vi "Write JSON Variant to File.vi"(8 "Error In":errorcluster, 10 "file (use dialog)":path, 11 "JSON Varaint":variant) -> (0 "error out":errorcluster)   [LabVIEW 2015]
uses:
  <vilib>/addons/_JKI.lib/Serialization/JSON/JKI JSON Serialization.lvlib
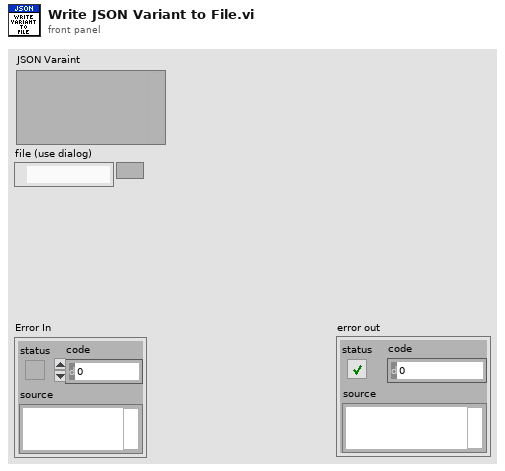
[diagram p1: front panel]
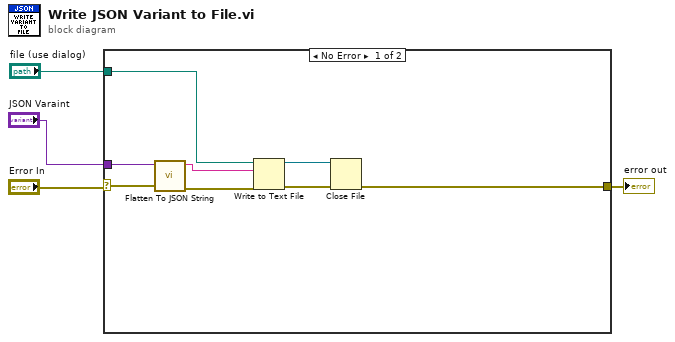
[diagram p0: block diagram]
diagram:
  n1 = case shown="No Error" "Error In" {
    selector: "Error In" -> [w12 w13]
    tunnel: "JSON Varaint" -> [w11 _]
    tunnel: "file (use dialog)" -> [w9 _]
    tunnel: [w5 w13] -> w1
    frame No Error {
      n2 = call <vilib>:"Flatten To JSON String.vi"("error in (no error)"=w12, "Variant"=w11) -> ("error out"=w10:errorcluster, "JSON String"=w8:string)  [unwired: 8 in]
      n3 = Write to Text File(file (use dialog)=w9, text=w8, error in=w10) -> (refnum out=w7:refnum<file>, error out=w6:errorcluster)  [unwired: 1 in, 1 out]
      n4 = Close File(refnum=w7, error in=w6) -> (error out=w5:errorcluster)  [unwired: 1 out]
    }
    frame Error {
    }
  }
  "error out" <- w1
